vi "azura_ScalableMultiFitSelectMODEL.vi"(3 "output control":T1, 4 "data":T2, 5 "x":dbl[](array[numeric]), 6 "a":dbl[](array[numeric])) -> (0 "error out":errorcluster, 1 "f'(X,a)":dbl[][](array[numeric]), 2 "f(X, a)":dbl[](array[numeric]))   [LabVIEW 2019]
doc: "This template is the starting point for creating a model function to be passed to the Nonlinear Curve Fit.vi."
uses:
  <vilib>/gmath/NumericalOptimization/objective function data.ctl
  <vilib>/gmath/NumericalOptimization/LM_output select.ctl
  <vilib>/gmath/NI_Gmath.lvlib
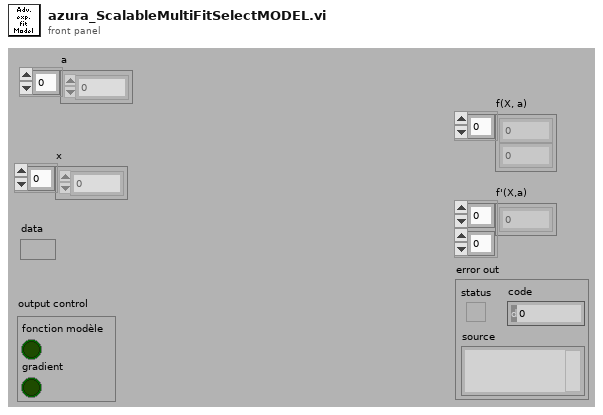
[diagram p1: front panel]
types:
  T1 = typedef "NI_Gmath.lvlib/LM_output select.ctl" = cluster{"model function":bool, "gradient":bool}
  T2 = typedef "NI_Gmath.lvlib/objective function data.ctl" = variant
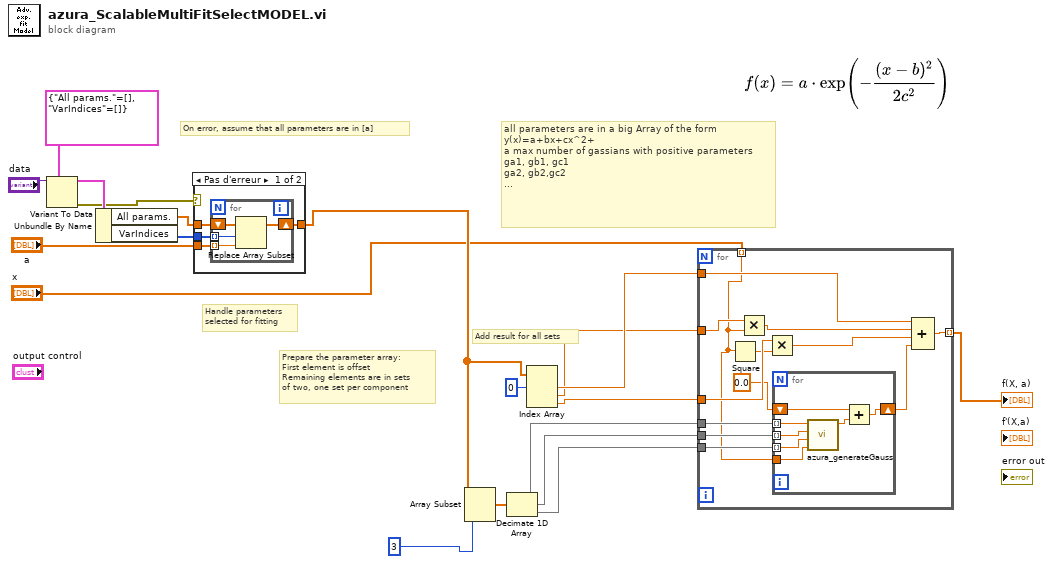
[diagram p0: block diagram]
diagram:
  # "all parameters are in a big Array of the form\ny(x)=a+bx+cx^2+\na max number of gassians with positive parameters\nga1, gb1, gc1\nga2, gb2,gc2\n..."
  # "On error, assume that all parameters are in [a]"
  # "Add result for all sets"
  # "Prepare the parameter array:\nFirst element is offset\nRemaining elements are in sets\nof two, one set per component"
  # "Handle parameters\nselected for fitting"
  n1 = Variant To Data(type=cluster{"All params.":dbl[], "VarIndices":i32[]} {"All params."=[], "VarIndices"=[]}, Variant="data") -> (data=w16:cluster{"All params.":dbl[], "VarIndices":i32[]}, error out=w13:errorcluster)  [unwired: 1 in]
  n2 = Unbundle By Name(w16) -> ("All params."=w14:dbl[], "VarIndices"=w15:i32[])
  n3 = case shown="Pas d'erreur" w13 {
    tunnel: "a" -> [w23 w28]
    tunnel: [w22 w28] -> w9
    tunnel: w14 -> [w21 _]
    tunnel: w15 -> [w20 _]
    frame No Error {
      n4 = for {
        shift-right: [w27] -> w22
        shift-left: w21 -> [w26]
        tunnel: w23 -> [w25] mode=indexing
        tunnel: w20 -> [w24] mode=indexing
        n5 = Replace Array Subset(array=w26, new element=w25, index=w24) -> (w27:dbl[])
      }
    }
    frame Error {
    }
  }
  n6 = Array Subset(array=w9, index=3 ("indice")) -> (w11:dbl[])  [unwired: 1 in]
  n7 = Decimate 1D Array(w11) -> (w5:dbl[], w4:dbl[], w3:dbl[])
  n8 = Index Array(array=w9, index #1=0 ("indice")) -> (element #1=w8:dbl, element #2=w7:dbl, element #3=w6:dbl)  [unwired: 2 in]
  n9 = for {
    tunnel: w7 -> [w39]
    tunnel: "x" -> [w29] mode=indexing
    tunnel: w6 -> [w37]
    tunnel: w5 -> [w34]
    tunnel: w4 -> [w33]
    tunnel: w3 -> [w32]
    tunnel: w8 -> [w40]
    tunnel: [w41] -> w1 mode=indexing
    n10 = Square(x=w29) -> (x^2=w36:dbl)
    n11 = Multiply(x=w39, y=w29) -> (x*y=w38:dbl)
    n12 = Multiply(x=w37, y=w36) -> (x*y=w35:dbl)
    n13 = for {
      tunnel: w34 -> [w48] mode=indexing
      tunnel: w33 -> [w47] mode=indexing
      tunnel: w32 -> [w46] mode=indexing
      tunnel: w29 -> [w45]
      shift-right: [w43] -> w30
      shift-left: 0.0 -> [w42]
      n14 = call "azura_generateGauss.vi"("x"=w45, "gc"=w46, "gb"=w47, "ga"=w48) -> ("f(x)"=w44:dbl)  [unwired: 7 in]
      n15 = Add(x=w42, y=w44) -> (x+y=w43:dbl)
    }
    n16 = Compound Arithmetic op=ADD(w40, w38, w35, w30) -> (w41:dbl)
  }
  "f(X, a)" <- w1
